vi "Value Change.vi"(5 "object ref in":T2, 8 "error in":errorcluster, 9 "old values":string[][](array[string]), 10 "Cluster":T1, 11 "String Column in":refnum<class "String Column.lvclass">) -> (0 "error out":errorcluster, 3 "String Column out":refnum<class "String Column.lvclass">)   [LabVIEW 2013, in "Table Manager.lvlib" / "String Column.lvclass"]
uses:
  String Column.lvclass
  Column/Column.lvclass
  <vilib>/NI/Tag Bus Data Framework/Configuration Editor/Classes/Engine Parent/Engine Parent Editor Node.lvclass
  <vilib>/NI/Tag Bus Data Framework/Configuration Editor/Classes/Module editor node/module editor node.lvclass
  Table Manager/object ref.ctl
  Table Manager/Table Manager.lvclass
  Table Manager/Cell Change.ctl
  Table Manager.lvlib
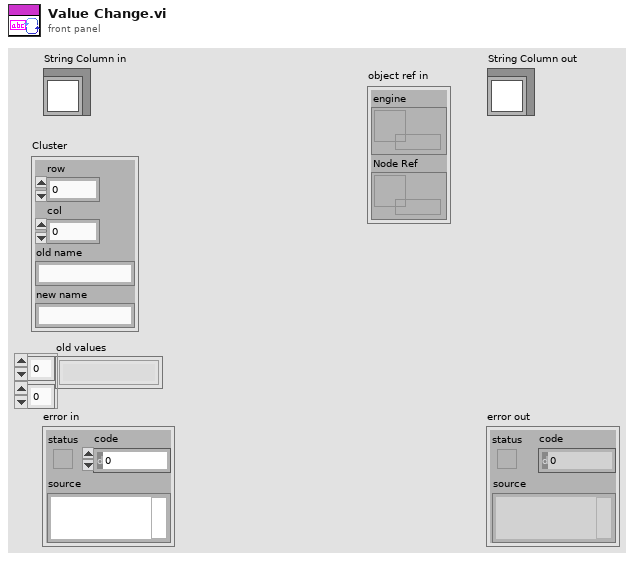
[diagram p1: front panel]
types:
  T1 = typedef "Table Manager.lvlib/Cell Change.ctl" = cluster{"row":i32, "col":i32, "old name":string, "new name":string}
  T2 = typedef "Table Manager.lvlib/Table Manager.lvclass/object ref.ctl" = cluster{"engine":refnum<data-value>, "Node Ref":refnum<data-value>}
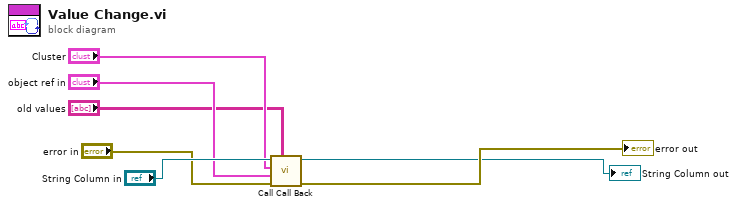
[diagram p0: block diagram]
diagram:
  n1 = call "Call Call Back.vi"("old values"="old values", "error in (no error)"="error in", "object ref in"="object ref in", "Table Change"="Cluster", "Column in"="String Column in") -> ("error out"=→"error out":errorcluster, "Column Out"=→"String Column out":refnum<class "String Column.lvclass">)  [unwired: 5 in]
